vi "CreateBlockDiagramImage.vi"(7 "Enum":enum16{"BD", "FP"}(ring), 8 "error (in)":errorcluster, 10 "JSON Path":path, 11 "VI in":refnum<vi>) -> (0 "error (out)":errorcluster, 1 "Image Path":path, 2 "Created Folder":path, 3 "Diagram out":refnum<vi>, 4 "MasterRect":T1)   [LabVIEW 2017]
doc: "Creates an image for block diagram\n1. Create destination folder for block diagram components\n2. Generate image"
uses:
  <vilib>/Utility/miscctls.llb/LVRectTypeDef.ctl
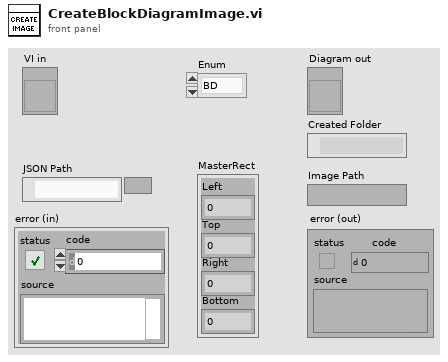
[diagram p1: front panel]
types:
  T1 = typedef "LVRectTypeDef.ctl" = cluster{"Left":i16, "Top":i16, "Right":i16, "Bottom":i16}
  T2 = typedef "imagedata.ctl" = cluster{"image type":i32, "image depth":i32, "image":u8[], "mask":u8[], "colors":u32[], "Rectangle":cluster{"left":i16, "top":i16, "right":i16, "bottom":i16}}
  T3 = cluster{"left":i16, "top":i16, "right":i16, "bottom":i16}
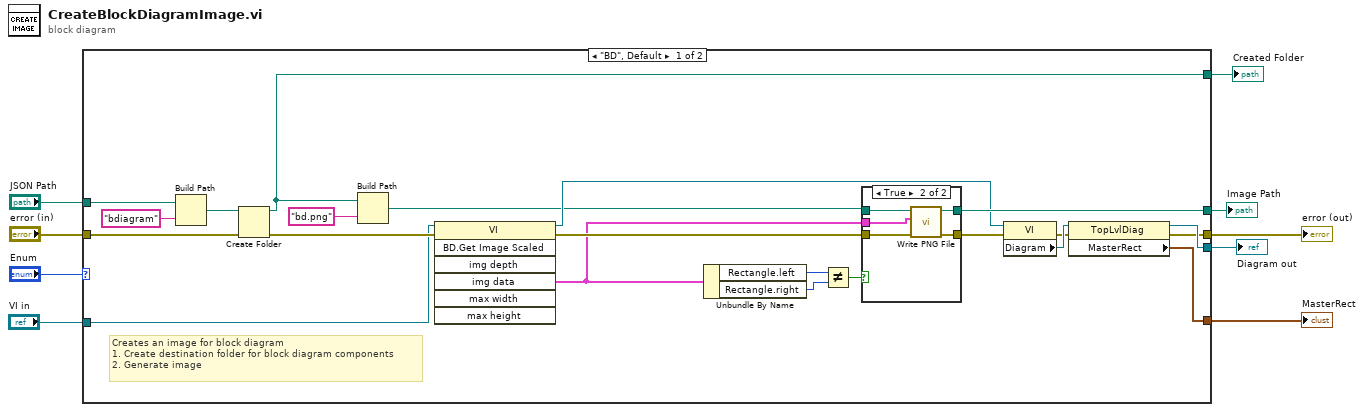
[diagram p0: block diagram]
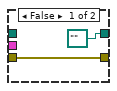
[diagram p2: hidden frame]
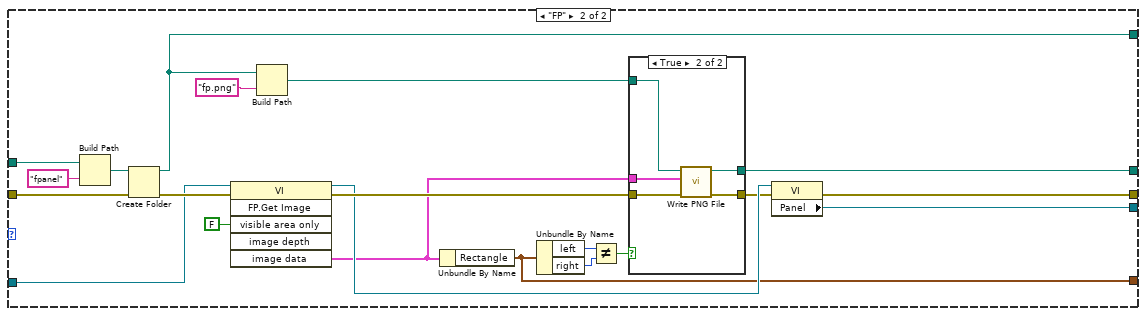
[diagram p3: hidden frame]
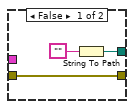
[diagram p4: hidden frame]
diagram:
  n1 = case shown="\"BD\", Default" "Enum" {
    tunnel: [w29 w57] -> w9
    tunnel: [w20 w52] -> w8
    tunnel: [w23 w51] -> w7
    tunnel: "JSON Path" -> [w14 w44]
    tunnel: "VI in" -> [w27 w56]
    tunnel: "error (in)" -> [w26 w55]
    tunnel: [w10 w40] -> w3
    tunnel: [w22 w48] -> w1
    frame "BD", Default {
      # "Creates an image for block diagram\n1. Create destination folder for block diagram components\n2. Generate image"
      n2 = Build Path(base path=w14, name or relative path="bdiagram" ("string")) -> (appended path=w13:path)
      n3 = Create Folder(path (use dialog)=w13, error in=w26) -> (created path=w10:path, error out=w31:errorcluster)  [unwired: 1 in, 1 out]
      n4 = Build Path(base path=w10, name or relative path="bd.png" ("string")) -> (appended path=w11:path)
      n5 = invoke class="VI" method="BD.Get Image Scaled"(reference=w27, error in=w31) -> (reference out=w28:refnum<vi>, error out=w30:errorcluster, "img data"=w19:T2)  [unwired: 5 in, 4 out]
      n6 = Unbundle By Name(w19) -> ("Rectangle.left"=w18:i16, "Rectangle.right"=w17:i16)
      n7 = Not Equal?(x=w18, y=w17) -> (x != y?=w16:bool)
      n8 = case shown="True" w16 {
        tunnel: w11 -> [_ w38]
        tunnel: w30 -> [w33 w37]
        tunnel: [path "" w36] -> w29
        tunnel: [w33 w35] -> w25
        tunnel: w19 -> [_ w34]
        frame False {
        }
        frame True {
          n9 = call <vilib>:"Write PNG File.vi"("error in (no error)"=w37, "image data"=w34, "path to PNG file"=w38) -> ("error out"=w35:errorcluster, "path"=w36:path)  [unwired: 7 in]
        }
      }
      n10 = property class="VI"(reference=w28, error in=w25) -> (error out=w21:errorcluster, "Diagram"=w24:refnum<vi>)  [unwired: 1 out]
      n11 = property class="TopLvlDiag"(reference=w24, error in=w21) -> (reference out=w23:refnum<vi>, error out=w20:errorcluster, "MasterRect"=w22:T1)
    }
    frame "FP" {
      n12 = Build Path(base path=w44, name or relative path="fpanel" ("string")) -> (appended path=w42:path)
      n13 = Create Folder(path (use dialog)=w42, error in=w55) -> (created path=w40:path, error out=w59:errorcluster)  [unwired: 1 in, 1 out]
      n14 = invoke class="VI" method="FP.Get Image"(reference=w56, error in=w59, "visible area only"=FALSE ("Visible Area Only")) -> (reference out=w54:refnum<vi>, error out=w58:errorcluster, "image data"=w49:T2)  [unwired: 3 in, 3 out]
      n15 = Build Path(base path=w40, name or relative path="fp.png" ("string")) -> (appended path=w39:path)
      n16 = Unbundle By Name(w49) -> ("Rectangle"=w48:T3)
      n17 = Unbundle By Name(w48) -> ("left"=w47:i16, "right"=w46:i16)
      n18 = Not Equal?(x=w47, y=w46) -> (x != y?=w45:bool)
      n19 = case shown="True" w45 {
        tunnel: w39 -> [_ w67]
        tunnel: w58 -> [w60 w66]
        tunnel: [w62 w65] -> w57
        tunnel: [w60 w64] -> w53
        tunnel: w49 -> [_ w63]
        frame False {
          n20 = String To Path(string="") -> (path=w62:path)
        }
        frame True {
          n21 = call <vilib>:"Write PNG File.vi"("error in (no error)"=w66, "image data"=w63, "path to PNG file"=w67) -> ("error out"=w64:errorcluster, "path"=w65:path)  [unwired: 7 in]
        }
      }
      n22 = property class="VI"(reference=w54, error in=w53) -> (error out=w52:errorcluster, "Panel"=w51:refnum<vi>)  [unwired: 1 out]
    }
  }
  "Diagram out" <- w7
  "Image Path" <- w9
  "error (out)" <- w8
  "Created Folder" <- w3
  "MasterRect" <- w1
